vi "LV SciSDK REGISTER FILE GET REGISTER.vi"(0 "Register Name":string, 7 "Register File Handle In":T2, 9 "Board Handle In":T1, 11 "error in (no error)":errorcluster) -> (4 "NI Error Code":i32, 6 "Register Value Out":i32, 8 "Register File Handle Out":T2, 10 "Board Handle Out":T1, 15 "error out":errorcluster)   [LabVIEW 2021, in "SciSDK_Labview.lvlib"]
doc: "You need this VI to get the value of a register that is inside a register file"
uses:
  SciSDK_Labview.lvlib
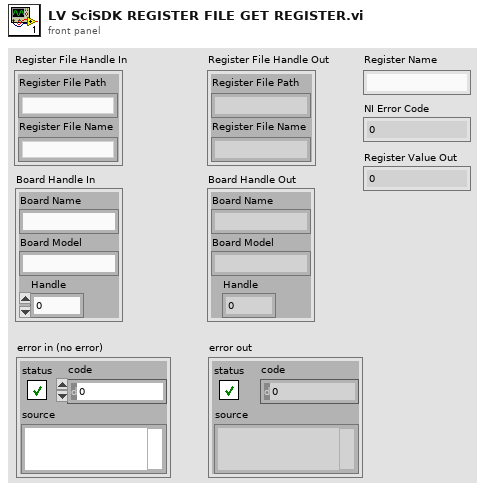
[diagram p1: front panel]
types:
  T1 = cluster{"Board Name":string, "Board Model":string, "Handle":u64}
  T2 = cluster{"Register File Path":string, "Register File Name":string}
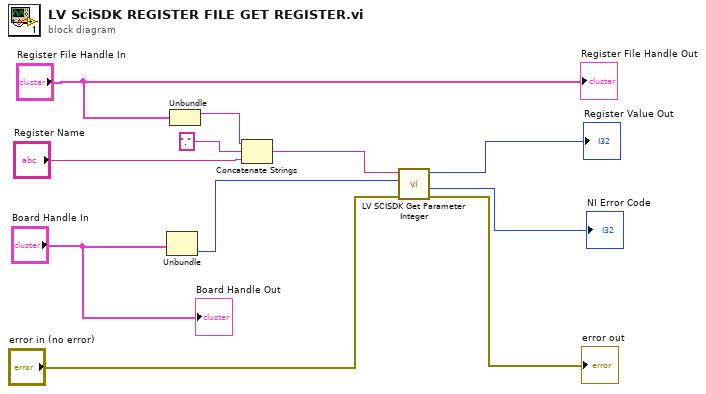
[diagram p0: block diagram]
diagram:
  n1 = Unbundle("Board Handle In") -> ("Handle"=w4:u64)  [unwired: 2 out]
  n2 = Unbundle("Register File Handle In") -> ("Register File Path"=w5:string)  [unwired: 1 out]
  n3 = Concatenate Strings(w5, "." ("string"), "Register Name") -> (w8:string)
  n4 = call "LV SCISDK Get Parameter Integer.vi"("error in (no error)"="error in (no error)", "handle"=w4, "Path"=w8) -> ("error out"=→"error out":errorcluster, "function return"=→"NI Error Code":i32, "value"=→"Register Value Out":i32)  [unwired: 5 in, 1 out]
  "Register File Handle Out" <- "Register File Handle In"
  "Board Handle Out" <- "Board Handle In"
